vi "Arr_OrCheck.vi"(1 "数组":u8[](array[numeric])) -> (0 "抑或的数据值":u8 format="%x")   [LabVIEW 2018]
panel:
  out "大小":i32
  out "数组 4":i32[](array[numeric]) format="%x"
  out "数组 3":i32[](array[numeric]) format="%x"
  out "数据值":u8 format="%x"
  out "数组 2":u8[](array[numeric]) format="%x"
  # "1"
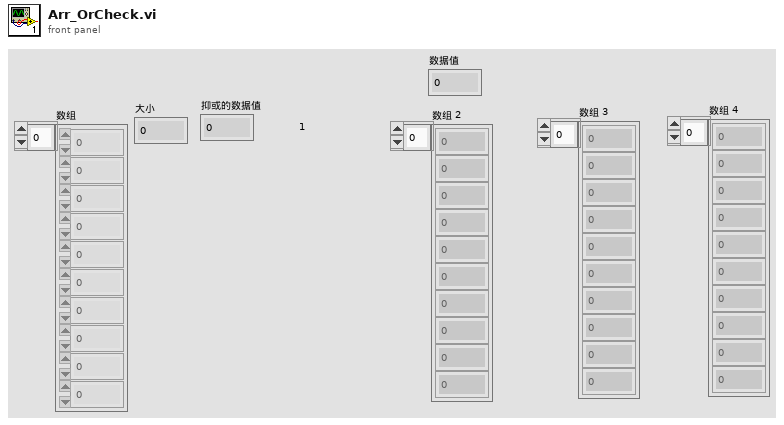
[diagram p1: front panel]
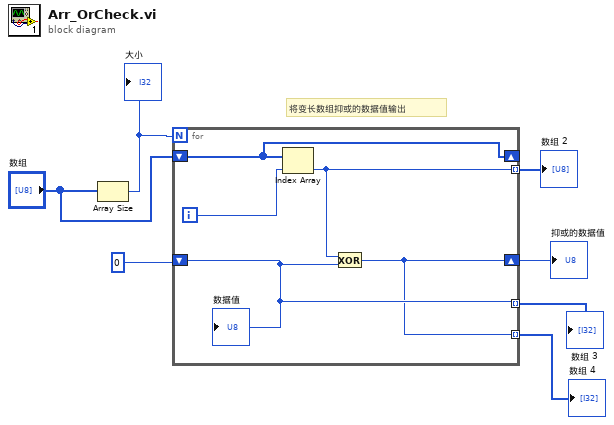
[diagram p0: block diagram]
diagram:
  # "将变长数组抑或的数据值输出"
  n1 = Array Size(array="数组") -> (size(s)=w7:i32)
  "大小" <- w7
  n2 = for {
    N: w7 -> [_]
    tunnel: [w12] -> w6 mode=indexing
    shift-right: [w9] -> w5
    shift-left: 0 -> [w10]
    tunnel: [w10] -> w3 mode=indexing
    tunnel: [w9] -> w2 mode=indexing
    shift-right: [w8] -> _
    shift-left: "数组" -> [w8]
    i -> [w11]
    n3 = Index Array(array=w8, index=w11) -> (element=w12:u8)
    n4 = Exclusive Or(1:w10, 2:w12) -> (0:w9:i32)
    "数据值" <- w10
  }
  "数组 2" <- w6
  "抑或的数据值" <- w5
  "数组 3" <- w3
  "数组 4" <- w2
